vi "Add Channel - System Storage.vi"(7 "GUID (Default Channel)":string="03D3BB99-1485-13A6-561D1F898F032919", 8 "error in (no error)":errorcluster, 9 "Channel":T2, 10 "Channel Name":string, 11 "Parent Ref in":T1 format="%.0x") -> (0 "error out":errorcluster, 1 "Channel Ref":T1 format="%.0x", 2 "Newly Created?":bool, 3 "Parent Ref out":T1 format="%.0x")   [LabVIEW 2011, in "Engine Sim System Explorer.lvlib"]
uses:
  <vilib>/NI Veristand/Custom Device API/Custom Device Item Ref.ctl
  <vilib>/NI Veristand/Custom Device API/Custom Device Channel.ctl
  <vilib>/NI Veristand/Custom Device API/Custom Device Channel Type.ctl
  NationalInstruments.VeriStand.SystemStorage
  Engine Sim System Explorer.lvlib
  <vilib>/NI Veristand/Custom Device API/Custom Device API.lvlib
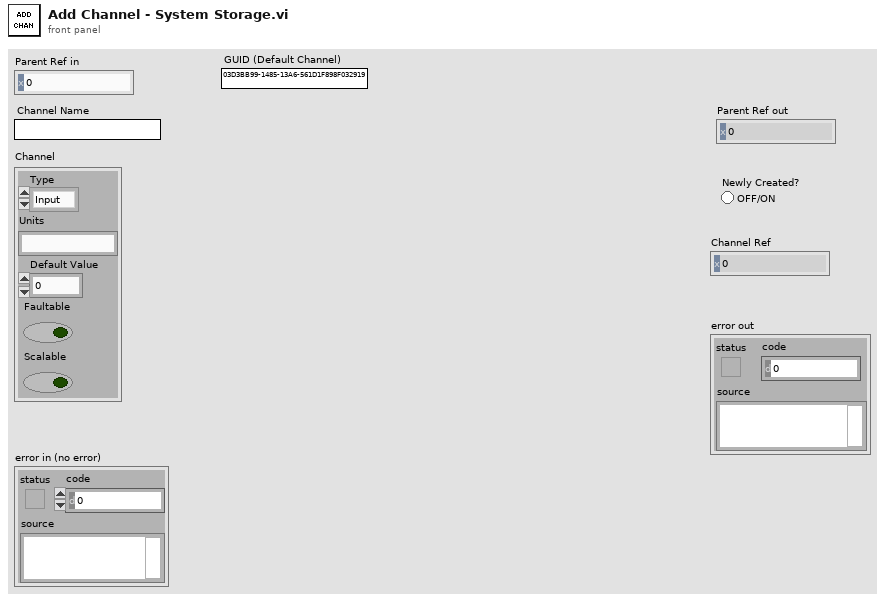
[diagram p1: front panel]
types:
  T1 = typedef "Custom Device API.lvlib/Custom Device Item Ref.ctl" = u64
  T2 = typedef "Custom Device API.lvlib/Custom Device Channel.ctl" = cluster{"Type":T3, "Units":string, "Default Value":dbl, "Faultable":bool, "Scalable":bool}
  T3 = typedef "Custom Device API.lvlib/Custom Device Channel Type.ctl" = enum16{"Input", "Output"}
  T4 = typedef "Custom Device API.lvlib/Custom Device Pointer.ctl" = refnum<k24>
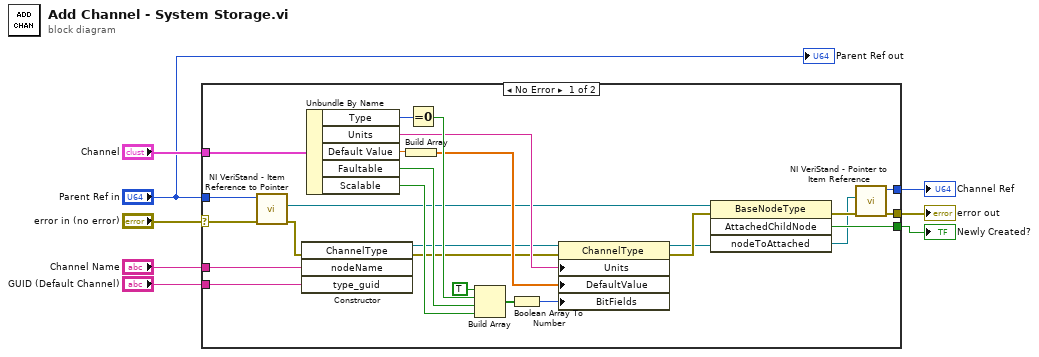
[diagram p0: block diagram]
diagram:
  n1 = case shown="No Error" "error in (no error)" {
    selector: "error in (no error)" -> [w33 w34]
    tunnel: "Parent Ref in" -> [w32 _]
    tunnel: "Channel Name" -> [w30 _]
    tunnel: "GUID (Default Channel)" -> [w29 _]
    tunnel: "Channel" -> [w28 _]
    tunnel: [w15 _] -> w2
    tunnel: [w10 w34] -> w3
    tunnel: [w14 _] -> w1
    frame No Error {
      n2 = call <vilib>:"NI VeriStand - Item Reference to Pointer.vi"("error in (no error)"=w33, "Item Ref in"=w32) -> ("error out"=w31:errorcluster, "Node Pointer"=w13:T4)  [unwired: 6 in, 2 out]
      n3 = constructor class="ChannelType"(error in=w31, "nodeName"=w30, "type_guid"=w29) -> (reference out=w17:refnum<k24>, error out=w16:errorcluster)  [unwired: 2 in, 3 out]
      n4 = Unbundle By Name(w28) -> ("Type"=w25:T3, "Units"=w20:string, "Default Value"=w19:dbl, "Faultable"=w26:bool, "Scalable"=w27:bool)
      n5 = Build Array(w19) -> (w18:dbl[])
      n6 = Equal To 0?(x=w25) -> (x = 0?=w24:bool)
      n7 = Build Array(TRUE ("element"), w24, w26, w27) -> (w22:bool[])
      n8 = Boolean Array To Number(Boolean array=w22) -> (number=w21:u32)
      n9 = property class="ChannelType"(reference=w17, error in=w16, "Units"=w20, "DefaultValue"=w18, "BitFields"=w21) -> (reference out=w9:refnum<k24>, error out=w12:errorcluster)
      n10 = invoke class="BaseNodeType" method="AttachedChildNode"(reference=w13, error in=w12, "nodeToAttached"=w9) -> (error out=w11:errorcluster, "AttachedChildNode"=w15:bool)  [unwired: 1 in, 2 out]
      n11 = call <vilib>:"NI VeriStand - Pointer to Item Reference.vi"("error in (no error)"=w11, "Node Pointer"=w9) -> ("error out"=w10:errorcluster, "Item Ref out"=w14:T1)  [unwired: 8 in]
    }
    frame Error {
    }
  }
  "Newly Created?" <- w2
  "Channel Ref" <- w1
  "error out" <- w3
  "Parent Ref out" <- "Parent Ref in"
